vi "Safety Variable.vi"() -> ()   [LabVIEW 2010]
panel:
  in  "Safety":dbl[](array[numeric])
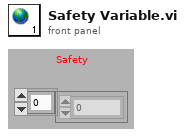
[diagram p1: front panel]
diagram:
